vi "Write Current.vi"(8 "error in":errorcluster, 10 "Current":dbl, 11 "57XX in":refnum<class "57XX.lvclass">) -> (0 "error out":errorcluster, 3 "57XX out":refnum<class "57XX.lvclass">)   [LabVIEW 2019, in "57XX.lvlib" / "57XX.lvclass"]
uses:
  Library/57XX.lvclass
  builds/Instruments/PowerSupply.lvlibp/Library/PowerSupply.lvclass
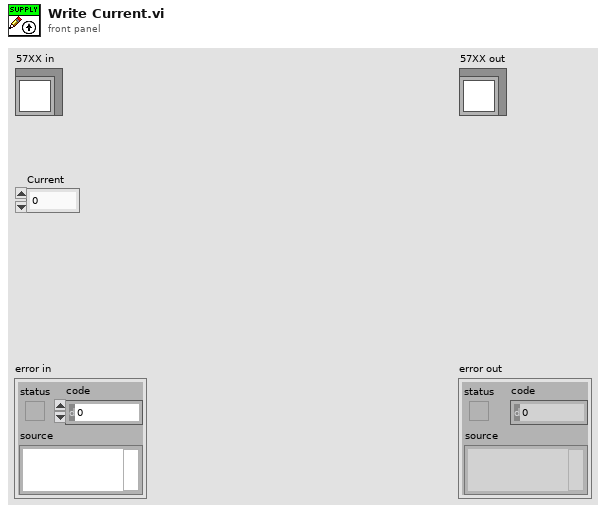
[diagram p1: front panel]
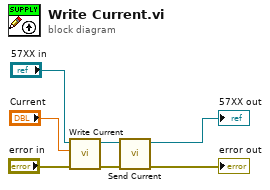
[diagram p0: block diagram]
diagram:
  n1 = call-parent "Write Current.vi"("error in"="error in", "Current"="Current", "PowerSupply in"="57XX in") -> ("error out"=w3:errorcluster, "PowerSupply out"=w4:refnum<class "57XX.lvclass">)  [unwired: 7 in]
  n2 = call "Send Current.vi"("error in (no error)"=w3, "57XX in"=w4) -> ("error out"=→"error out":errorcluster, "57XX out"=→"57XX out":refnum<class "57XX.lvclass">)  [unwired: 8 in]
